vi "GLIMPSE Launcher.vi"() -> ()   [LabVIEW 2015]
doc: "The main menu for GLIMPSE. Click the buttons to activate different program features."
uses:
  GLIMPSE Globals.vi
panel:
  in  "Run Plug-ins":bool
  in  "About Glimpse":bool
  in  "Delete acquisition files":bool
  in  "Defunct VCR Batch Acquire":bool
  in  "Filter":bool
  in  "Subtract background":bool
  in  "Save to other format":bool
  in  "Read from other format":bool
  in  "Generate Test Sequence":bool
  in  "Help Window":bool
  in  "Frame skipping test":bool
  in  "Play sequence/Track Objects":bool
  in  "Playback/Save Mode":T1(ring)
  in  "Exit":bool
  # "Test/debug tools"
  # "Sequence Files"
  # "View Sequence"
  # "Process"
  # "Control Program"
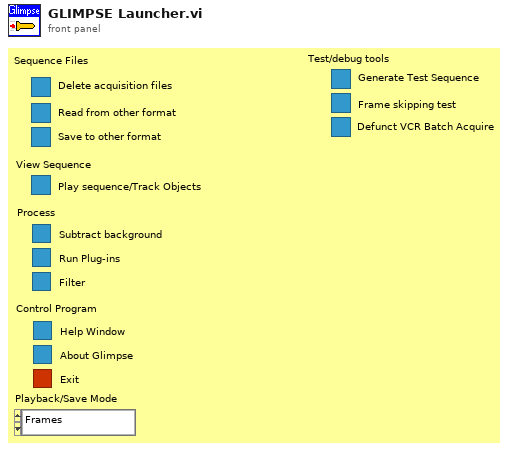
[diagram p1: front panel]
types:
  T1 = enum16{"Frames", "Fields, Odd 1st", "Fields, Even 1st", "Fields, Averaged"}
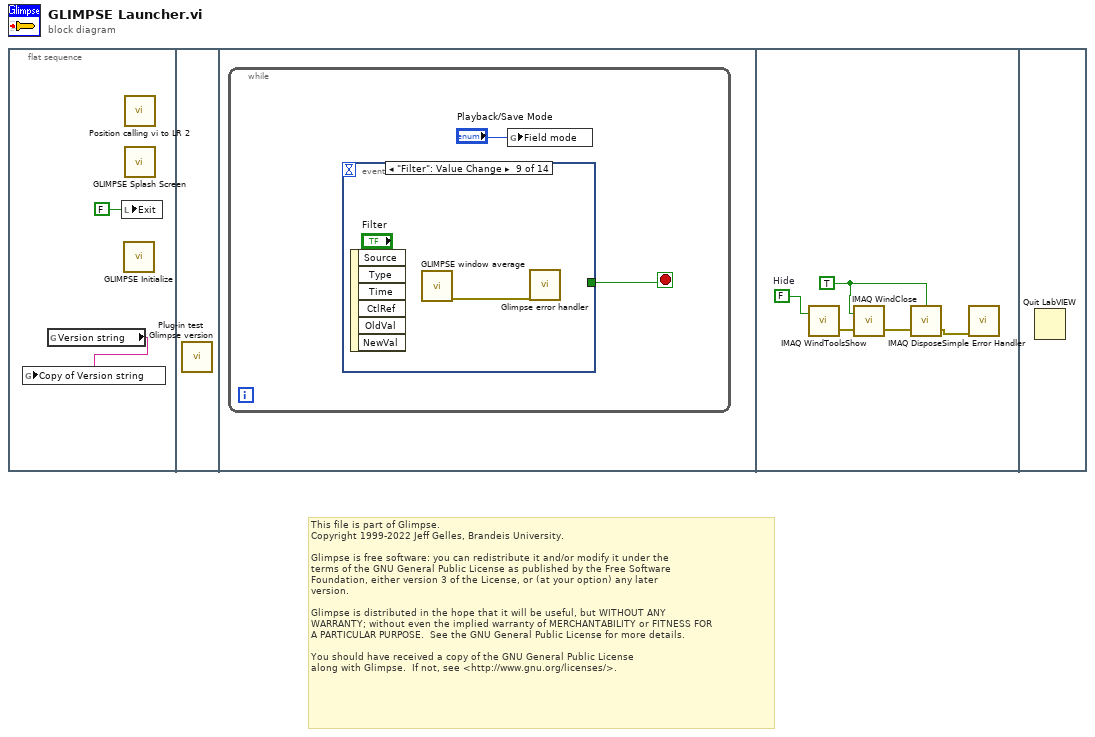
[diagram p0: block diagram]
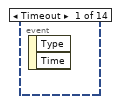
[diagram p2: hidden frame]
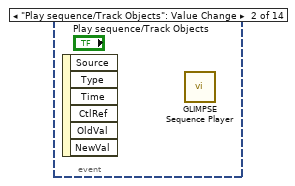
[diagram p3: hidden frame]
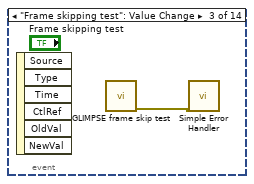
[diagram p4: hidden frame]
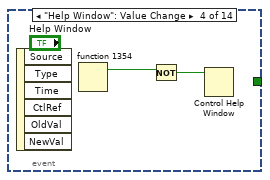
[diagram p5: hidden frame]
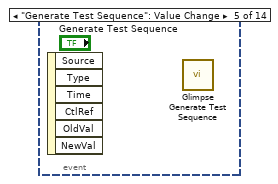
[diagram p6: hidden frame]
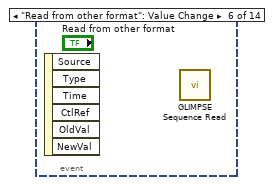
[diagram p7: hidden frame]
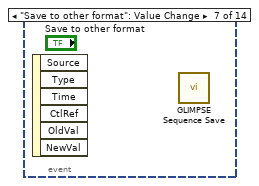
[diagram p8: hidden frame]
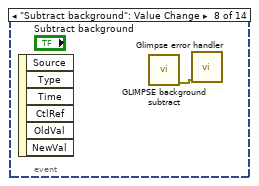
[diagram p9: hidden frame]
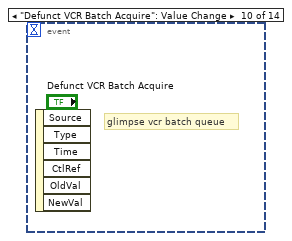
[diagram p10: hidden frame]
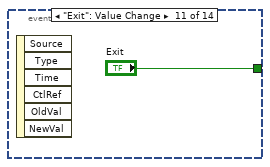
[diagram p11: hidden frame]
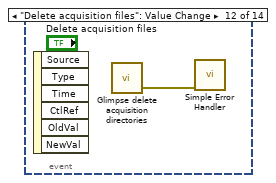
[diagram p12: hidden frame]
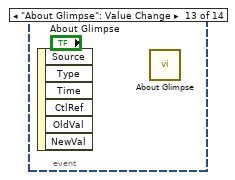
[diagram p13: hidden frame]
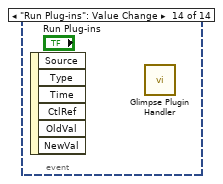
[diagram p14: hidden frame]
diagram:
  # "This file is part of Glimpse. \nCopyright 1999-2022 Jeff Gelles, Brandeis University.    \n\nGlimpse is free software: you can redistribute it and/or modify it under the \nterms of the GNU General Public License as published by the Free Software \nFoundation, either version 3 of the License, or (at your option) any later \nversion.\n\nGlimpse is distributed in the hope that it will be useful, but WITHOUT ANY \nWARRANTY; without even the implied warranty of MERCHANTABILITY or FITNESS FOR \nA PARTICULAR PURPOSE.  See the GNU General Public License for more details.\n\nYou should have received a copy of the GNU General Public License\nalong with Glimpse.  If not, see <http://www.gnu.org/licenses/>."
  n1 = flat-sequence {
    frame #0 {
      n2 = global read "GLIMPSE Globals.vi" "Version string"() -> (w1:string)
      n3 = global write "GLIMPSE Globals.vi" "Copy of Version string"(w1) -> ()
      n4 = local write "Exit"(FALSE ("Exit")) -> ()
      n5 = call "GLIMPSE Initialize.vi"() -> ()  [unwired: 10 out]
      n6 = call "Position calling vi to LR 2.vi"() -> ()  [unwired: 2 in, 4 out]
      n7 = call "GLIMPSE Splash Screen.vi"() -> ()  [unwired: 1 out]
    }
    frame #1 {
      n8 = call "Plug-in test Glimpse version.vi"() -> ()  [unwired: 1 in, 7 out]
    }
    frame #2 {
      n9 = while {
        stop <- w3 stop-if-true
        n10 = event shown="[8] \"Filter\": Value Change" {
          selector: _ -> [_ _ _ _ _ _ _ _ _ _ _ _ _ _]
          dyn-events: _ -> [_ _ _ _ _ _ _ _ _ _ _ _ _ _]
          timeout: _ -> [_ _ _ _ _ _ _ _ _ _ _ _ _ _]
          tunnel: [_ _ _ _ _ _ _ _ _ _ "Exit" _ _ _] -> w3
          event Timeout {
            n11 = event-data() -> ()  [unwired: 3 out]
          }
          event "Play sequence/Track Objects": Value Change {
            n12 = event-data() -> ()  [unwired: 7 out]
            n13 = call "GLIMPSE Sequence Player.vi"() -> ()  [unwired: 1 in, 8 out]
          }
          event "Frame skipping test": Value Change {
            n14 = event-data() -> ()  [unwired: 7 out]
            n15 = call "GLIMPSE frame skip test.vi"() -> ("error out"=w5:errorcluster)  [unwired: 1 in, 6 out]
            n16 = call <vilib>:"Simple Error Handler.vi"("error in (no error)"=w5) -> ()  [unwired: 1 in, 8 out]
          }
          event "Help Window": Value Change {
            n17 = event-data() -> ()  [unwired: 7 out]
            n18 = fn#1354() -> (1:w6:bool)  [unwired: 1 out]
            n19 = Not(x=w6) -> (.not. x?=w7:bool)
            n20 = Control Help Window(1:w7) -> ()  [unwired: 1 out]
          }
          event "Generate Test Sequence": Value Change {
            n21 = event-data() -> ()  [unwired: 7 out]
            n22 = call "Glimpse Generate Test Sequence.vi"() -> ()  [unwired: 1 out]
          }
          event "Read from other format": Value Change {
            n23 = event-data() -> ()  [unwired: 7 out]
            n24 = call "GLIMPSE Sequence Read.vi"() -> ()  [unwired: 1 out]
          }
          event "Save to other format": Value Change {
            n25 = event-data() -> ()  [unwired: 7 out]
            n26 = call "GLIMPSE Sequence Save.vi"() -> ()  [unwired: 4 in, 6 out]
          }
          event "Subtract background": Value Change {
            n27 = event-data() -> ()  [unwired: 7 out]
            n28 = call "GLIMPSE background subtract.vi"() -> ("error out"=w8:errorcluster)  [unwired: 5 in, 5 out]
            n29 = call "Glimpse error handler.vi"("error in"=w8) -> ()  [unwired: 1 in, 6 out]
          }
          event "Filter": Value Change {
            n30 = event-data() -> ()  [unwired: 7 out]
            n31 = call "GLIMPSE window average.vi"() -> ("error out"=w9:errorcluster)  [unwired: 2 in, 5 out]
            n32 = call "Glimpse error handler.vi"("error in"=w9) -> ()  [unwired: 1 in, 6 out]
          }
          event "Defunct VCR Batch Acquire": Value Change {
            # "glimpse vcr batch queue"
            n33 = event-data() -> ()  [unwired: 7 out]
          }
          event "Exit": Value Change {
            n34 = event-data() -> ()  [unwired: 7 out]
          }
          event "Delete acquisition files": Value Change {
            n35 = event-data() -> ()  [unwired: 7 out]
            n36 = call "Glimpse delete acquisition directories.vi"() -> ("error out"=w11:errorcluster)  [unwired: 1 in, 6 out]
            n37 = call <vilib>:"Simple Error Handler.vi"("error in (no error)"=w11) -> ()  [unwired: 1 in, 8 out]
          }
          event "About Glimpse": Value Change {
            n38 = event-data() -> ()  [unwired: 7 out]
            n39 = call "About Glimpse.vi"() -> ()  [unwired: 1 out]
          }
          event "Run Plug-ins": Value Change {
            n40 = event-data() -> ()  [unwired: 7 out]
            n41 = call "Glimpse Plugin Handler.vi"() -> ()  [unwired: 1 out]
          }
        }
        n42 = global write "GLIMPSE Globals.vi" "Field mode"("Playback/Save Mode") -> ()
      }
    }
    frame #3 {
      w12 = TRUE ("All Images? (No)")
      w16 = FALSE  # Hide
      n43 = call "IMAQ WindToolsShow"("Hide/Show (Show)"=w16) -> ("error out"=w15:errorcluster)  [unwired: 2 in, 3 out]
      n44 = call "IMAQ WindClose"("Close All Windows (False)"=w12, "error in (no error)"=w15) -> ("error out"=w13:errorcluster)  [unwired: 1 in, 3 out]
      n45 = call "IMAQ Dispose"("All Images? (No)"=w12, "error in (no error)"=w13) -> ("error out"=w14:errorcluster)  [unwired: 1 in, 3 out]
      n46 = call <vilib>:"Simple Error Handler.vi"("error in (no error)"=w14) -> ()  [unwired: 1 in, 8 out]
    }
    frame #4 {
      n47 = Quit LabVIEW() -> ()  [unwired: 1 out]
    }
  }
